vi "sv_Set Chirp Waveform Attributes.vi"(8 "error in (no error)":errorcluster, 10 "chirp settings":T1={"amplitude"=1.0, "frequency range"={"start (Hz)"=20.0, "stop (Hz)"=20000.0, "frequency spacing"=enum."Logarithmic"}, "sampling info"={"Fs"=50000.0, "chirp duration [s]"=3.0}, "initial states"={"frequency [Hz]"=20.0, "phase [rad]"=0.0, "elapsed time [s]"=0.0}, "frequency slope"=0.0, "maximum harmonic"=3, "prefix len [samples]"={"integer"=0, "fractional"=0.0}} {"frequency slope" format="%.2f"; "prefix len [samples]"."fractional" format="%.2p"; "initial states"."elapsed time [s]" format="%.2f"; "initial states"."phase [rad]" format="%.2f"; "initial states"."frequency [Hz]" format="%.2f"; "sampling info"."chirp duration [s]" format="%.2f"; "sampling info"."Fs" format="%.2p"; "frequency range"."stop (Hz)" format="%.2f"; "frequency range"."start (Hz)" format="%.2f"; "amplitude" format="%.2f"}, 11 "chirp signal":waveform(dbl)={"t0"=timestamp(0 s since 1904-01-01), "dt"=0.0, "Y"=[]}) -> (0 "error out":errorcluster, 3 "chirp signal out":waveform(dbl))   [LabVIEW 2017, in "SoundVib_Generation.lvlib"]
uses:
  <vilib>/addons/_NISVFA/_Generation/SoundVib_Generation.lvlib
  <vilib>/addons/_NISVFA/_Generation/subVIs/sv_Chirp Settings.ctl
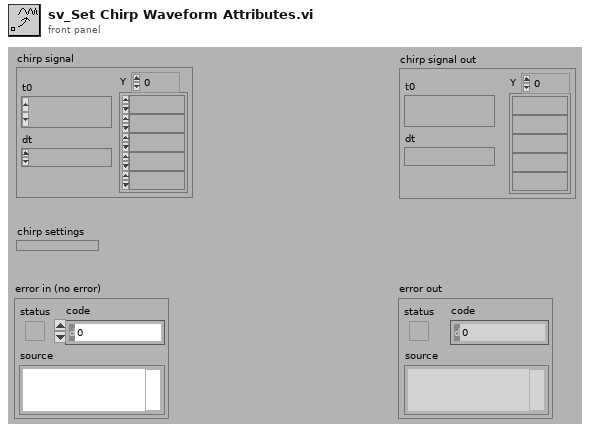
[diagram p1: front panel]
types:
  T1 = typedef "SoundVib_Generation.lvlib/sv_Chirp Settings.ctl" = cluster{"amplitude":dbl, "frequency range":cluster{"start (Hz)":dbl, "stop (Hz)":dbl, "frequency spacing":enum16{"Linear", "Logarithmic"}}, "sampling info":cluster{"Fs":dbl, "chirp duration [s]":dbl}, "initial states":cluster{"frequency [Hz]":dbl, "phase [rad]":dbl, "elapsed time [s]":dbl}, "frequency slope":dbl, "maximum harmonic":i32, "prefix len [samples]":cluster{"integer":u32, "fractional":dbl}}
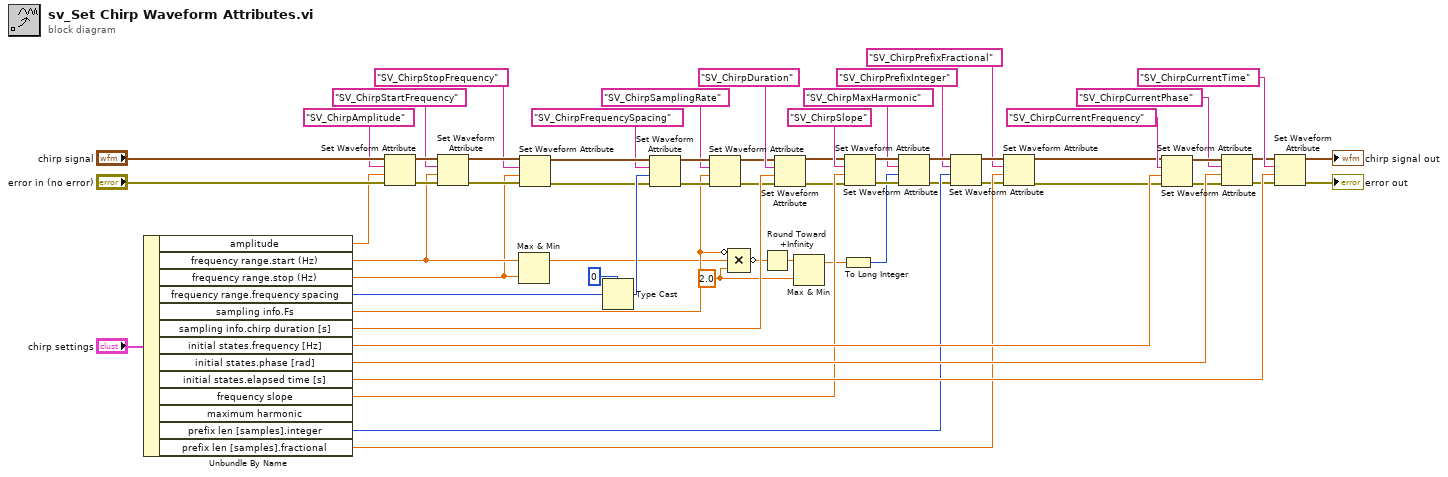
[diagram p0: block diagram]
diagram:
  w7 = 2.0 ("value")
  n1 = Unbundle By Name("chirp settings") -> ("amplitude"=w57:dbl, "frequency range.start (Hz)"=w5:dbl, "frequency range.stop (Hz)"=w4:dbl, "frequency range.frequency spacing"=w49:enum16{"Linear", "Logarithmic"}, "sampling info.Fs"=w6:dbl, "sampling info.chirp duration [s]"=w56:dbl, "initial states.frequency [Hz]"=w55:dbl, "initial states.phase [rad]"=w54:dbl, "initial states.elapsed time [s]"=w53:dbl, "frequency slope"=w52:dbl, "prefix len [samples].integer"=w51:u32, "prefix len [samples].fractional"=w50:dbl)  [unwired: 1 out]
  n2 = Set Waveform Attribute(4:"error in (no error)", 5:w57, 6:"SV_ChirpAmplitude" ("name"), 7:"chirp signal") -> (0:w35:errorcluster, 3:w36:waveform(dbl))  [unwired: 1 out]
  n3 = Set Waveform Attribute(4:w35, 5:w5, 6:"SV_ChirpStartFrequency" ("name"), 7:w36) -> (0:w32:errorcluster, 3:w33:waveform(dbl))  [unwired: 1 out]
  n4 = Max & Min(x=w5, y=w4) -> (max(x,y)=w3:dbl)  [unwired: 1 out]
  n5 = Set Waveform Attribute(4:w32, 5:w4, 6:"SV_ChirpStopFrequency" ("name"), 7:w33) -> (0:w30:errorcluster, 3:w29:waveform(dbl))  [unwired: 1 out]
  n6 = Type Cast(type=u16 0, x=w49) -> (*(type *) &x=w47:u16)
  n7 = Set Waveform Attribute(4:w30, 5:w47, 6:"SV_ChirpFrequencySpacing" ("name"), 7:w29) -> (0:w26:errorcluster, 3:w27:waveform(dbl))  [unwired: 1 out]
  n8 = Set Waveform Attribute(4:w26, 5:w6, 6:"SV_ChirpSamplingRate" ("name"), 7:w27) -> (0:w12:errorcluster, 3:w13:waveform(dbl))  [unwired: 1 out]
  n9 = Compound Arithmetic op=MULTIPLY(invert w6, w3, w7) -> (invert w9:dbl)
  n10 = Round Toward +Infinity(x=w9) -> (ceil(x): smallest int >= x=w8:dbl)
  n11 = Set Waveform Attribute(4:w12, 5:w56, 6:"SV_ChirpDuration" ("name"), 7:w13) -> (0:w10:errorcluster, 3:w11:waveform(dbl))  [unwired: 1 out]
  n12 = Max & Min(x=w8, y=w7) -> (max(x,y)=w2:dbl)  [unwired: 1 out]
  n13 = To Long Integer(number=w2) -> (32bit integer=w1:i32)
  n14 = Set Waveform Attribute(4:w10, 5:w52, 6:"SV_ChirpSlope" ("name"), 7:w11) -> (0:w21:errorcluster, 3:w22:waveform(dbl))  [unwired: 1 out]
  n15 = Set Waveform Attribute(4:w21, 5:w1, 6:"SV_ChirpMaxHarmonic" ("name"), 7:w22) -> (0:w18:errorcluster, 3:w19:waveform(dbl))  [unwired: 1 out]
  n16 = Set Waveform Attribute(4:w18, 5:w51, 6:"SV_ChirpPrefixInteger" ("name"), 7:w19) -> (0:w15:errorcluster, 3:w16:waveform(dbl))  [unwired: 1 out]
  n17 = Set Waveform Attribute(4:w15, 5:w50, 6:"SV_ChirpPrefixFractional" ("name"), 7:w16) -> (0:w39:errorcluster, 3:w38:waveform(dbl))  [unwired: 1 out]
  n18 = Set Waveform Attribute(4:w39, 5:w55, 6:"SV_ChirpCurrentFrequency" ("name"), 7:w38) -> (0:w45:errorcluster, 3:w44:waveform(dbl))  [unwired: 1 out]
  n19 = Set Waveform Attribute(4:w45, 5:w54, 6:"SV_ChirpCurrentPhase" ("name"), 7:w44) -> (0:w40:errorcluster, 3:w41:waveform(dbl))  [unwired: 1 out]
  n20 = Set Waveform Attribute(4:w40, 5:w53, 6:"SV_ChirpCurrentTime" ("name"), 7:w41) -> (0:→"error out":errorcluster, 3:→"chirp signal out":waveform(dbl))  [unwired: 1 out]
